vi "Exponential Smooth.vi"(10 "Smoothing Factor":dbl=0.1, 11 "Input Value":dbl) -> (3 "Smoothed Value":dbl)   [LabVIEW 2011]
doc: "Exponential smoothing weights the input value against the previous smoothing value."
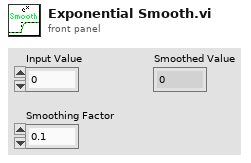
[diagram p1: front panel]
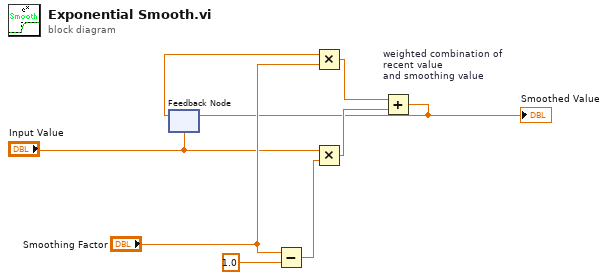
[diagram p0: block diagram]
diagram:
  n1 = feedback #1("Input Value") -> (w2:dbl)
  n2 = Subtract(x="Smoothing Factor", y=1.0) -> (x-y=w8:dbl)
  n3 = Multiply(x=w2, y="Smoothing Factor") -> (x*y=w1:dbl)
  n4 = Multiply(x="Input Value", y=w8) -> (x*y=w5:dbl)
  n5 = Add "weighted combination of\nrecent value\nand smoothing value"(x=w1, y=w5) -> (x+y=w4:dbl)
  "Smoothed Value" <- w4
  n6 = feedback-in #1(w4) -> ()
